vi "Condition Msg VI.vi"(8 "error in":errorcluster, 10 "Ref.Msg VI":refnum<vi>) -> (0 "error out":errorcluster)   [LabVIEW 2020, in "_Msg Rescript.lvlib" / "_Msg Rescript.lvclass"]
uses:
  _Msg Rescript.lvclass
  <vilib>/Utility/traverseref.llb/TRef TravTarget.ctl
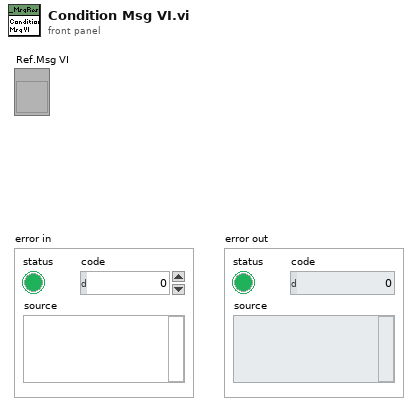
[diagram p1: front panel]
types:
  T1 = typedef "TRef TravTarget.ctl" = enum16{"FP", "BD", "Other"}
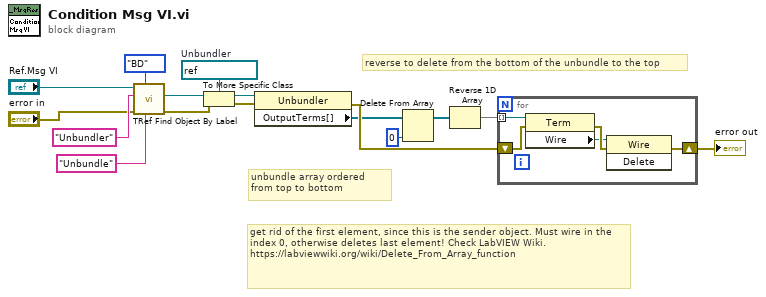
[diagram p0: block diagram]
diagram:
  w14 = refnum<vi> refnum  # Unbundler
  # "reverse to delete from the bottom of the unbundle to the top"
  # "unbundle array ordered from top to bottom"
  # "get rid of the first element, since this is the sender object. Must wire in the index 0, otherwise deletes last element! Check LabVIEW Wiki.\nhttps://labviewwiki.org/wiki/Delete_From_Array_function"
  n1 = call <vilib>:"TRef Find Object By Label.vi"("Label"="Unbundle", "Traverse Target"=TRef_TravTarget."BD", "error in (no error)"="error in", "Class Name"="Unbundler", "VI Ref"="Ref.Msg VI") -> ("error out"=w15:errorcluster, "Found Obj Ref"=w13:refnum<vi>)  [unwired: 3 in, 2 out]
  n2 = To More Specific Class(target class=w14, reference=w13, error in=w15) -> (specific class reference=w10:refnum<vi>, error out=w8:errorcluster)
  n3 = property class="Unbundler"(reference=w10, error in=w8) -> (error out=w16:errorcluster, "OutputTerms[]"=w7:refnum<vi>[])  [unwired: 1 out]
  n4 = Delete From Array(array=w7, index=0) -> (array with subset deleted=w5:refnum<vi>[])  [unwired: 1 in, 1 out]
  n5 = Reverse 1D Array(array=w5) -> (reversed array=w1:refnum<vi>[])
  n6 = for {
    shift-right: [w17] -> w2
    shift-left: w16 -> [w18]
    tunnel: w1 -> [w20] mode=indexing
    n7 = property class="Term"(reference=w20, error in=w18) -> (error out=w21:errorcluster, "Wire"=w19:refnum<vi>)  [unwired: 1 out]
    n8 = invoke class="Wire" method="Delete"(reference=w19, error in=w21) -> (error out=w17:errorcluster)  [unwired: 1 in, 2 out]
  }
  "error out" <- w2
